vi "Turn LED ON.vi"() -> (3 "Boolean":bool=TRUE)   [LabVIEW 2020]
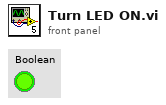
[diagram p1: front panel]
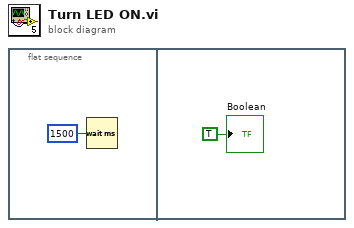
[diagram p0: block diagram]
diagram:
  n1 = flat-sequence {
    frame #0 {
      n2 = Wait (ms)(milliseconds to wait=u32 1500) -> ()  [unwired: 1 out]
    }
    frame #1 {
      "Boolean" <- TRUE
    }
  }
